vi "filteredCentroid.vi"(0 "image":T1, 5 "percentOffset":dbl=0.33, 9 "errorIn":errorcluster, 11 "imageArray":u16[][](array[numeric])) -> (4 "imageMasked":T1, 6 "Centroid":cluster{"X Centroid":sgl, "Y Centroid":sgl} {"Y Centroid" format="%.2f"; "X Centroid" format="%.2f"}, 10 "minMax":u16[](array[numeric]), 15 "errorOut":errorcluster)   [LabVIEW 2021]
uses:
  <vilib>/vision/Image Controls.llb/IMAQ Image.ctl
  <vilib>/vision/NI_Vision_Development_Module.lvlib
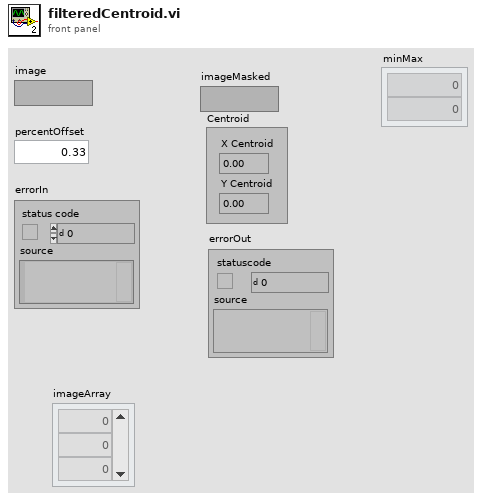
[diagram p1: front panel]
types:
  T1 = typedef "IMAQ Image.ctl" = refnum<image>
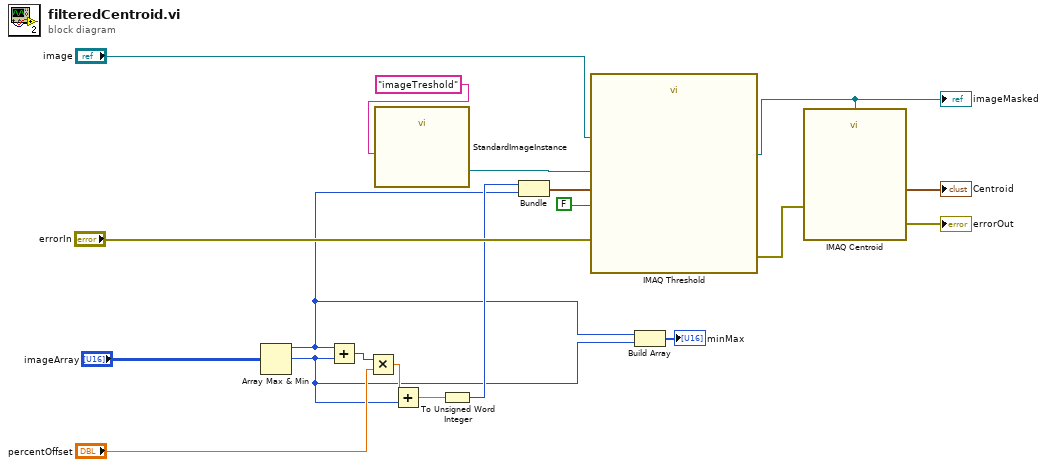
[diagram p0: block diagram]
diagram:
  n1 = Array Max & Min(array="imageArray") -> (max value=w4:u16, min value=w3:u16)  [unwired: 2 out]
  n2 = Add(x=w4, y=w3) -> (x+y=w16:u16)
  n3 = Multiply(x=w16, y="percentOffset") -> (x*y=w15:dbl)
  n4 = call "StandardImageInstance.vi"("Image Name"="imageTreshold") -> ("Refnum out"=w11:T1)  [unwired: 10 in]
  n5 = Add(x=w15, y=w3) -> (x+y=w7:dbl)
  n6 = To Unsigned Word Integer(number=w7) -> (unsigned 16bit integer=w6:u16)
  n7 = Bundle(w6, w4) -> (w5:cluster{u16, u16})  [unwired: 1 in]
  n8 = call "IMAQ Threshold"("Keep/Replace Value (Replace)"=FALSE, "error in (no error)"="errorIn", "Range"=w5, "Image Dst"=w11, "Image Src"="image") -> ("error out"=w8:errorcluster, "Image Dst Out"=w9:T1)  [unwired: 5 in]
  "imageMasked" <- w9
  n9 = Build Array(w4, w3) -> (→"minMax":u16[])
  n10 = call "IMAQ Centroid"("error in (no error)"=w8, "Image"=w9) -> ("error out"=→"errorOut":errorcluster, "Centroid"=→"Centroid":cluster{"X Centroid":sgl, "Y Centroid":sgl})  [unwired: 2 in]
